vi "STATE_machine_exp.vi"() -> ()   [LabVIEW 2019]
uses:
  A-Z.ctl
panel:
  out "String":string
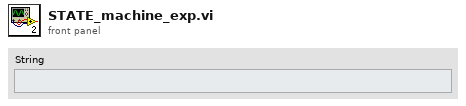
[diagram p1: front panel]
types:
  T1 = typedef "A-Z.ctl" = i32
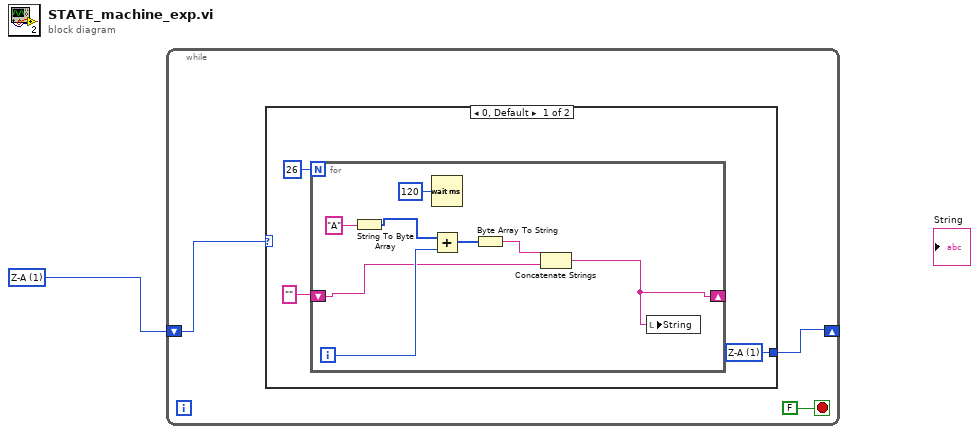
[diagram p0: block diagram]
diagram:
  w1 = T1 1 items=["A-Z", "Z-A"] ("Text Ring")
  n1 = while {
    shift-right: [w3] -> _
    shift-left: w1 -> [w4]
    stop <- FALSE stop-if-true
    n2 = case shown="0, Default" w4 {
      tunnel: [w5 _] -> w3
      frame 0, Default {
        w5 = T1 1 items=["A-Z", "Z-A"] ("Text Ring")
        n3 = for {
          N: 26 -> [_]
          shift-right: [w8] -> _
          shift-left: "" -> [w10]
          i -> [w13]
          n4 = String To Byte Array(string="A") -> (unsigned byte array=w14:u8[])
          n5 = Wait (ms)(milliseconds to wait=u32 120) -> ()  [unwired: 1 out]
          n6 = Add(x=w14, y=w13) -> (x+y=w12:i32[])
          n7 = Byte Array To String(unsigned byte array=w12) -> (string=w11:string)
          n8 = Concatenate Strings(w11, w10) -> (w8:string)
          n9 = local write "String"(w8) -> ()
        }
      }
      frame 1 {
      }
    }
  }
